vi "FL3001_simple.VI"() -> ()   [LabVIEW 2015]
uses:
  board.vis/Globals.vi
  board.vis/ESLSCDLL.dll
panel:
  in  "refresh display":bool
  in  "exit":bool
  in  "Trig Input Sel":string(combo)="I"
  out "meanB":dbl=197.0 format="%0#.1f"
  out "tRMSB":dbl format="%0#.1f"
  out "meanA":dbl=5347.758620689655 format="%0#.1f"
  in  "TRMS Pix":u32=400
  out "Signal Cam 2":u16[](graph)
  in  "extTrig":bool
  in  "ext. trig. slope":enum32{"1", "2", "3"}(radio)
  out "tRMSA":dbl=3.3455635332332063 format="%0#.1f"
  out "Measure ON":bool
  in  "no.of blocks (nob)":u32=1
  in  "block":u32(slide)=1 max=10 scale=0.9..1.0
  out "Signal Board 1 / Cam1":u16[](graph)=[0, 0, 0, 1, 0, 1, 0, 0, 5497, 8570, 8917, 9054, 9014, 9011, 8998, 9036, 9115, 9126, 9247, 9215, 9246, 9218, 9274, 9317, 9288, 9273, 9333, 9364, 9336, 9444, 9291, 9321, 9410, 9473, 9505, 9572, 9432, 9485, 9538, 9474, 9597, 9570, 9529, 9555, 9568, 9553, 9543, 9482, 9667, 9586, 9609, 9646, 9700, 9684, 9610, 9559, 9714, 9684, 9600, 9717, 9720, 9617, 9735, 9735, 9735, 9706, 9735, 9735, 9724, 9648, 9727, 9727, 9651, 9658, 9703, 9711, 9697, 9735, 9710, 9735, 9871, 9735, 9735, 9735, 9735, 9735, 9735, 9735, 9720, 9735, 9735, 9876, 9735, 9734, 9718, 9735, 9735, 9735, 9735, 9896, 9870, 9735, 9735, 9735, 9735, 9735, 9735, 9731, 9932, 9735, 9728, 9735, 9933, 9917, 9680, 9735, 9913, 9735, 9735, 9735, 9735, 9735, 9735, 9735, 9735, 9900, 9735, 9735, 9735, 9735, 9735, 9735, 9735, 9735, 9735, 9735, 9735, 9891, 9735, 9869, 9735, 9735, 9735, 9735, 9735, 9735, 9735, 9735, 9735, 9735, 9902, 9735, 9735, 9735, 9735, 9732, 9735, 9735, 9735, 9735, 9735, 9894, 9735, 9875, 9735, 9735, 9735, 9735, 9735, 9735, 9735, 9925, 9934, 9735, 9735, 9735, 9735, 9877, 9735, 9894, 9894, 9735, 9735, 9890, 9735, 9963, 9947, 9883, 9735, 9735, 9735, 9735, 9898, 9927, 9926, 9952, 9735, 9900, 9735, 9938, 9735, 9999, 9977, 9896, 9978, 9903, 9992, 9940, 9965, 9972, 9735, 9974, 9735, 9943, 9873, 9890, 9951, 9735, 9964, 9735, 9992, 9918, 10003, 9919, 9973, 9735, 9896, 9896, 9735, 9940, 10059, 9926, 9897, 9961, 9968, 9915, 9880, 9916, 9991, 9981, 9735, 9978, 10057, 10022, 9951, 9912, 9969, 10066, 9928, 9946, 9951, 10004, 9935, 9910, 9960, 9921, 9967, 9908, 10022, 9955, 9950, 9962, 9962, 9978, 10000, 9945, 9940, 9978, 9986, 10047, 10095, 9939, 10007, 9948, 10071, 10018, 10092, 10027, 10006, 10025, 10016, 10008, 10045, 10094, 10057, 10015, 9980, 10003, 10025, 10019, 10014, 10103, 10047, 9995, 9975, 10138, 9958, 10025, 9965, 10086, 10022, 9960, 10109, 10037, 10043, 10076, 10012, 10010, 10040, 10037, 10000, 9996, 10090, 10132, 10050, 10050, 9991, 10116, 10059, 10020, 9985, 10079, 10137, 10064, 10103, 10043, 10005, 10137, 10107, 10092, 10078, 10139, 10116, 10148, 10041, 10091, 10039, 10069, 10046, 10113, 10119, 10079, 10014, 10045, 10124, 10112, 10080, 10078, 10067, 10093, 10156, 10161, 10131, 10151, 10111, 10118, 10100, 10072, 10153, 10172, 10163, 10113, 10125, 10187, 10213, 10211, 10146, 10170, 10120, 10172, 10077, 10186, 10108, 10147, 10099, 10127, 10161, 10114, 10109, 10218, 10209, 10174, 10156, 10147, 10098, 10193, 10177, 10190, 10185, 10147, 10180, 10135, 10151, 10144, 10173, 10482, 10205, 10182, 10105, 10207, 10215, 10147, 10122, 10147, 10188, 10187, 10297, 10207, 10115, 10233, 10231, 10246, 10236, 10256, 10271, 10232, 10232, 10198, 10175, 10232, 10564, 10282, 10222, 10134, 10340, 10253, 10266, 10312, 10194, 10208, 10153, 10194, 10218, 10179, 10251, 10242, 10262, 10234, 10211, 10210, 10229, 10205, 10227, 10211, 10268, 10255, 10212, 10295, 10243, 10248, 10300, 10201, 10225, 10298, 10255, 10352, 10304, 10240, 10334, 10327, 10325, 10300, 10276, 10265, 10364, 10398, 10298, 10265, 10342, 10319, 10332, 10280, 10334, 10259, 10289, 10320, 10273, 10294, 10427, 10387, 10281, 10324, 10324, 10315, 10335, 10341, 10321, 10380, 10352, 10293, 10355, 10423, 10374, 10308, 10329, 10401, 10279, 11416, 10373, 10318, 10310, 10350, 10286, 10333, 10303, 10281, 10363, 10329, 10276, 10327, 10356, 10393, 10437, 10417, 10337, 10389, 10438, 10363, 10291, 10454, 10447, 10266, 10322, 10409, 10343, 10389, 10407, 10326, 10380, 10378, 10322, 10335, 10361, 10312, 10329, 10343, 10401, 10350, 10362, 10352, 10347, 10372, 10402, 10407, 10402, 10361, 10404, 10384, 10493, 10339, 10430, 10429, 10334, 10457, 10394, 10379, 10345, 10409, 10433, 10512, 10454, 10403, 10368, 10445, 10364, 10434, 10509, 10467, 10453, 10407, 10414, 10461, 10399, 10459, 10476, 10405, 10418, 10429, 10467, 10393, 10461, 10499, 10439, 10483, 10451, 10436, 10372, 10445, 10481, 10491, 10448, 10435, 10510, 10509, 10512, 10476, 10470, 10419, 10469, 10508, 10515, 10514, 10463, 10510, 10507, 10527, 10416, 10465, 10444, 10437, 10510, 10525, 10459, 10409, 10578, 10533, 10509, 10581, 10555, 10621, 10511, 10513, 10488, 10466, 10587, 10601, 10603, 10494, 10519, 10575, 10460, 10496, 10545, 10455, 10502, 10542, 10475, 10456, 10469, 10566, 10452, 10576, 10513, 10643, 10552, 10556, 10544, 10479, 10519, 10544, 10437, 10576, 10474, 10585, 10417, 10545, 10643, 10477, 10506, 10460, 10539, 10587, 10643, 10549, 10524, 10502, 10496, 10534, 10537, 10530, 10582, 10618, 10512, 10494, 10586, 10528, 10518, 10577, 10547, 10557, 10679, 10436, 10617, 10585, 10485, 10610, 10678, 10567, 10497, 10495, 10553, 10677, 10554, 10617, 10623, 10617, 10547, 10583, 10650, 10704, 10558, 10628, 10619, 10568, 10576, 10520, 10595, 10589, 10614, 10460, 10593, 10615, 10565, 10627, 10590, 10643, 10583, 10526, 10589, 10603, 10598, 10578, 10606, 10647, 10516, 10522, 10601, 10689, 10687, 10606, 10572, 10684, 10640, 10579, 10535, 10597, 10627, 10623, 10582, 10553, 10609, 10619, 10613, 10686, 10680, 10604, 10555, 10513, 10531, 10709, 10633, 10611, 10573, 10665, 10752, 10626, 10715, 10690, 10633, 10665, 10631, 10588, 10582, 10660, 10647, 10663, 10649, 10658, 10619, 10558, 10617, 10608, 10657, 10649, 10651, 10626, 10630, 10619, 10720, 10702, 10608, 10656, 10663, 10651, 10739, 10599, 10751, 10614, 10660, 10665, 10635, 10597, 10682, 10635, 10625, 10619, 10729, 10601, 10661, 10693, 10647, 10695, 10687, 10646, 10677, 10745, 10663, 10624, 10662, 10698, 10658, 10675, 10590, 10626, 10689, 10665, 10702, 10649, 10656, 10597, 10729, 10699, 10665, 10739, 10668, 10656, 10697, 10671, 10754, 10633, 10681, 10705, 10725, 10664, 10621, 10703, 10759, 10720, 10759, 10659, 10759, 10750, 10703, 10712, 10698, 10712, 10669, 10663, 10741, 10729, 10731, 10723, 10641, 10699, 10654, 10674, 10653, 10663, 10703, 10724, 10657, 10746, 10738, 10709, 10724, 10759, 10759, 10682, 10655, 10692, 10716, 10699, 10670, 10722, 10697, 10633, 10650, 10759, 10699, 10672, 10755, 10726, 10753, 10664, 10630, 10712, 10697, 10720, 10759, 10744, 10704, 10759, 10721, 10661, 10747, 10656, 10680, 10645, 10671, 10716, 10647, 10709, 10738, 10756, 10683, 10650, 10656, 10605, 10557, 10656, 10638, 10597, 10587, 10589, 10596, 10551, 10586, 10613, 10549, 10648, 10610, 10570, 10644, 10618, 10658, 10588, 10583, 10591, 10618, 10599, 10492, 10557, 10493, 10465, 10580, 10506, 10559, 10531, 10541, 10518, 10495, 10514, 10612, 10520, 10539, 10503, 10568, 10606, 10536, 10503, 10525, 10512, 10524, 10471, 10493, 10519, 10619, 10517, 10491, 10560, 10479, 10575, 10449, 10491, 10502, 10527, 10519, 10465, 10521, 10457, 10404, 10530, 10450, 10445, 10454, 10491, 10424, 10471, 10480, 10435, 10423, 10556, 10465, 10497, 10507, 10400, 10511, 10498, 10429, 10429, 10548, 10503, 10437, 10482, 10473, 10435, 10423, 10438, 10414, 10409, 10345, 10391, 10570, 10351, 10411, 10503, 10555, 10309, 10345, 10368, 10407, 10394, 10398, 10418, 10394, 10348, 10377, 10290, 10358, 10383, 10359, 10398, 10280, 10223, 10349, 10302, 10359, 10281, 10282, 10260, 10188, 10223, 10184, 10210, 10173, 10175, 10143, 10053, 10065, 10066, 10009, 10013, 9955, 9944, 9883, 5845, 5634, 5619, 5774, 5415, 5385, 5374, 5370, 5361, 5366, 5361, 5359, 5363, 5356, 5359, 5362, 5357, 5358, 5359, 5358, 5357, 5355, 5363, 5369, 5359, 5359, 5361, 5362, 5362, 5361, 5363, 5362, 5359, 5365, 5358, 5366, 5364, 5356, 5356, 5360, 5359, 5363, 5362]
  out "FREE \nRAM MB":dbl=28847.8671875
  out "BUILT-IN\nRAM MB":dbl=32640.29296875
  out "SEC":dbl=1.0
  out "MB RAM":dbl=2.0751953125
  in  "DAT in 10ns":u32
  in  "start":bool
  in  "sample":u32(slide)=1 max=3000 scale=0.9..1000.0
  in  "no.of samples (nos)":u32=1000
  in  "exposuretime[ms]":dbl=1.0 format="%.3f"
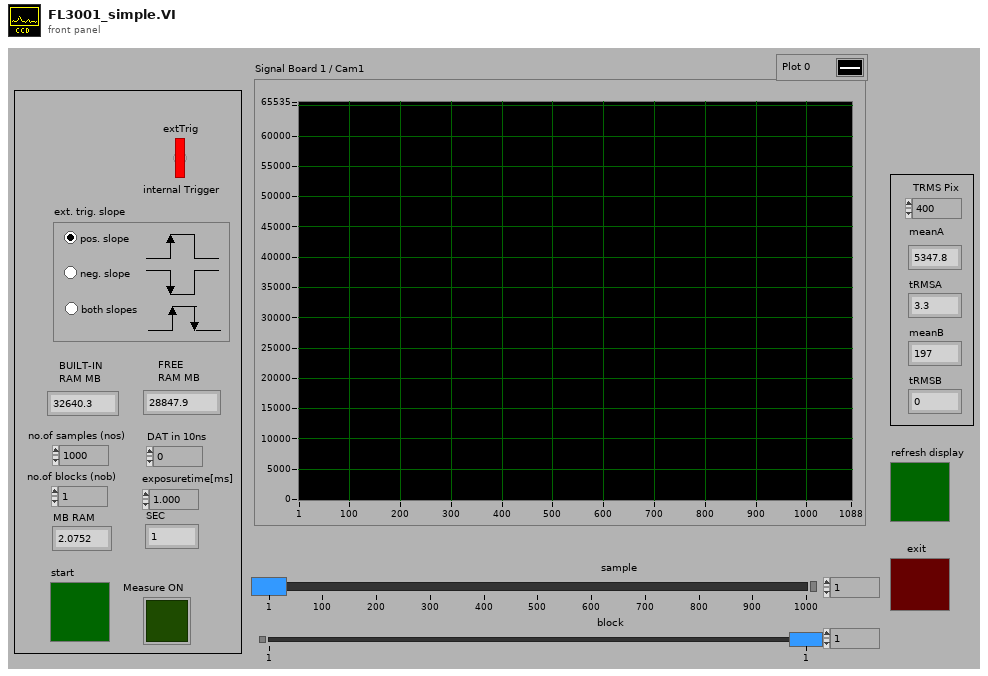
[diagram p1: front panel]
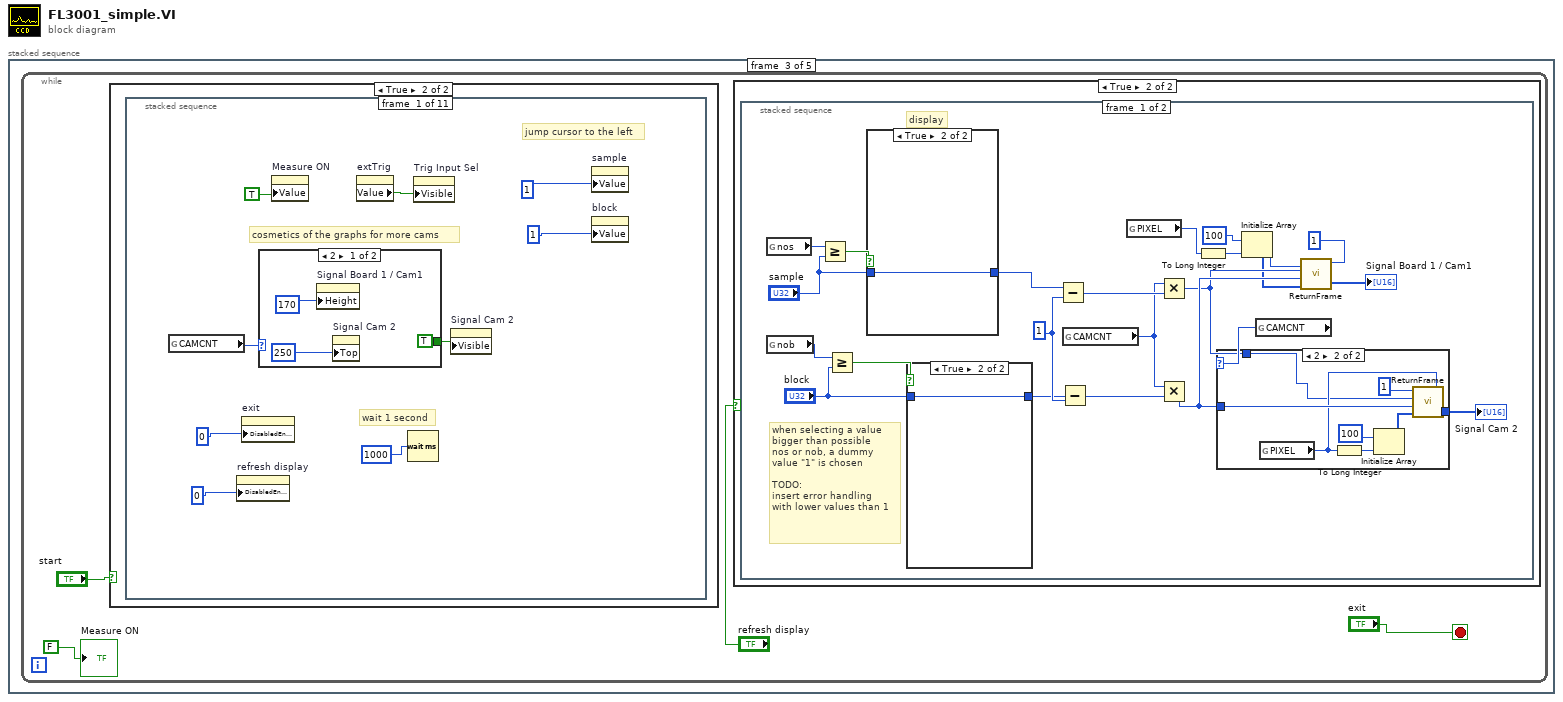
[diagram p0: block diagram]
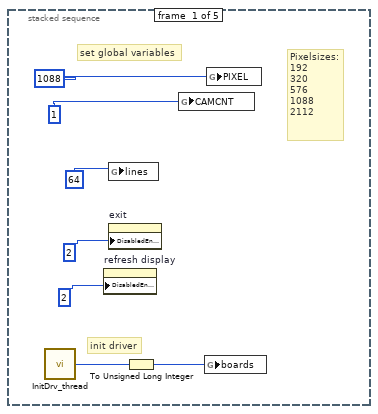
[diagram p2: hidden frame]
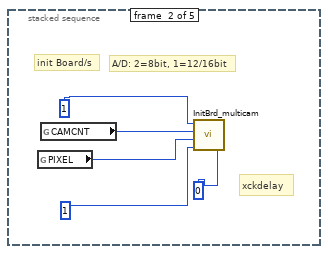
[diagram p3: hidden frame]
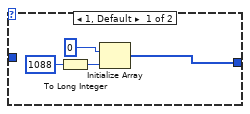
[diagram p5: hidden frame]
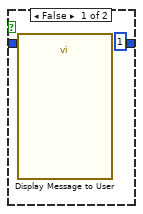
[diagram p6: hidden frame]
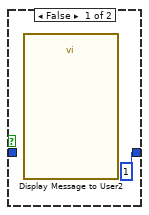
[diagram p7: hidden frame]
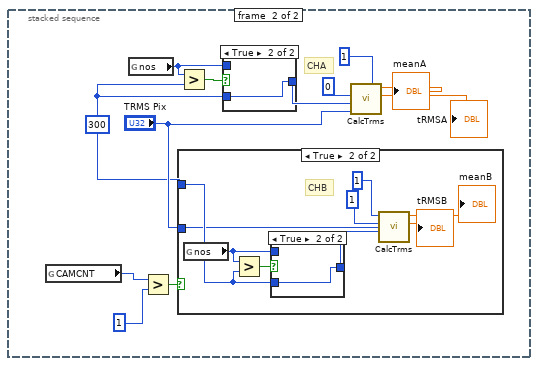
[diagram p8: hidden frame]
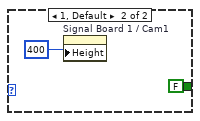
[diagram p13: hidden frame]
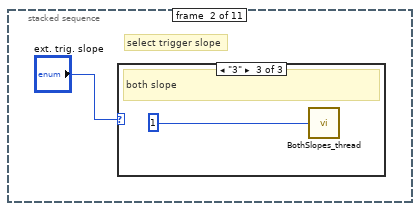
[diagram p14: hidden frame]
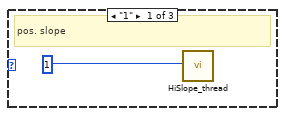
[diagram p15: hidden frame]
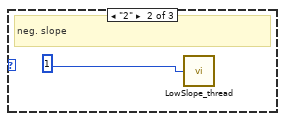
[diagram p16: hidden frame]
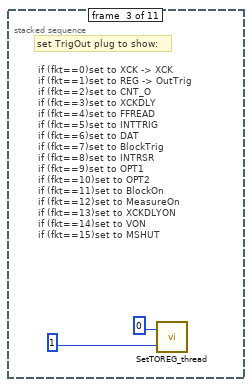
[diagram p17: hidden frame]
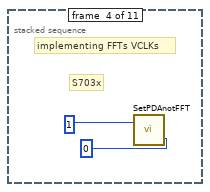
[diagram p18: hidden frame]
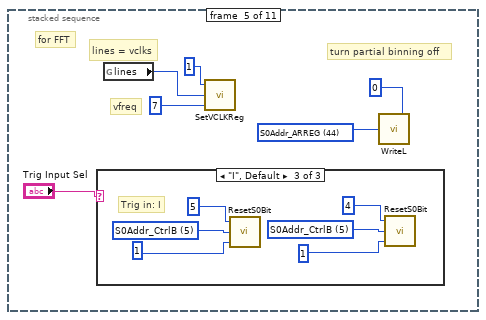
[diagram p19: hidden frame]
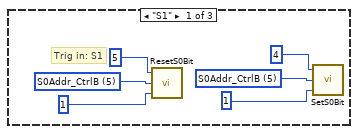
[diagram p20: hidden frame]
diagram:
  n1 = stacked-sequence {
    frame #0 {
      # "Pixelsizes:\n192\n320\n576\n1088\n2112"
      # "set global variables"
      # "init driver"
      n2 = call "InitDrv_thread.vi"() -> ("Boards"=w5:u8)  [unwired: 1 in]
      n3 = property on="refresh display" class="Bool (strict)"("DisabledEnum"=u16 2) -> ()  [unwired: 2 in, 2 out]
      n4 = global write "Globals.vi" "lines"(u32 64) -> ()
      n5 = property on="exit" class="Bool (strict)"("DisabledEnum"=u16 2) -> ()  [unwired: 2 in, 2 out]
      n6 = To Unsigned Long Integer(number=w5) -> (unsigned 32bit integer=w4:u32)
      n7 = global write "Globals.vi" "CAMCNT"(u32 1) -> ()
      n8 = global write "Globals.vi" "boards"(w4) -> ()
      n9 = global write "Globals.vi" "PIXEL"(u32 1088) -> ()
    }
    frame #1 {
      # "xckdelay"
      # "init Board/s"
      # "A/D: 2=8bit, 1=12/16bit"
      n10 = global read "Globals.vi" "PIXEL"() -> (w10:u32)
      n11 = global read "Globals.vi" "CAMCNT"() -> (w12:u32)
      n12 = call "InitBrd_multicam.vi"("xckdly"=u32 0, "flag816"=u32 1, "pixel"=w10, "camcnt"=w12, "board_sel"=u32 1) -> ()  [unwired: 2 in]
    }
    frame #2 {
      n13 = while {
        stop <- "exit" stop-if-true
        n14 = case shown="True" "start" {
          frame False {
          }
          frame True {
            n15 = stacked-sequence {
              frame #0 {
                # "wait 1 second"
                # "jump cursor to the left"
                # "cosmetics of the graphs for more cams"
                n16 = global read "Globals.vi" "CAMCNT"() -> (w87:u32)
                n17 = property on="refresh display" class="Bool (strict)"("DisabledEnum"=u16 0) -> ()  [unwired: 2 in, 2 out]
                n18 = property on="exit" class="Bool (strict)"("DisabledEnum"=u16 0) -> ()  [unwired: 2 in, 2 out]
                n19 = case shown="2" w87 {
                  tunnel: [TRUE FALSE] -> w88
                  frame 2 {
                    n20 = property on="Signal Board 1 / Cam1" class="WFGraph (strict)"("Height"=u32 170) -> ()  [unwired: 2 in, 2 out]
                    n21 = property on="Signal Cam 2" class="WFGraph (strict)"("Top"=250) -> ()  [unwired: 2 in, 2 out]
                  }
                  frame 1, Default {
                    n22 = property on="Signal Board 1 / Cam1" class="WFGraph (strict)"("Height"=u32 400) -> ()  [unwired: 2 in, 2 out]
                  }
                }
                n23 = property on="Measure ON" class="Bool (strict)"("Value"=TRUE) -> ()  [unwired: 2 in, 2 out]
                n24 = property on="extTrig" class="Bool (strict)"() -> ("Value"=w85:bool)  [unwired: 2 in, 2 out]
                n25 = Wait (ms)(milliseconds to wait=u16 1000) -> ()  [unwired: 1 out]
                n26 = property on="Trig Input Sel" class="CmbBox"("Visible"=w85) -> ()  [unwired: 2 in, 2 out]
                n27 = property on="Signal Cam 2" class="WFGraph (strict)"("Visible"=w88) -> ()  [unwired: 2 in, 2 out]
                n28 = property on="sample" class="Slide (strict)"("Value"=u32 1) -> ()  [unwired: 2 in, 2 out]
                n29 = property on="block" class="Slide (strict)"("Value"=u32 1) -> ()  [unwired: 2 in, 2 out]
              }
              frame #1 {
                # "select trigger slope"
                n30 = case shown="\"3\"" "ext. trig. slope" {
                  frame "1" {
                    # "pos. slope"
                    n31 = call "HiSlope_thread.vi"("board_sel"=u32 1) -> ()  [unwired: 1 in]
                  }
                  frame "2" {
                    # "neg. slope"
                    n32 = call "LowSlope_thread.vi"("board_sel"=u32 1) -> ()  [unwired: 1 in]
                  }
                  frame "3" {
                    # "both slope"
                    n33 = call "BothSlopes_thread.vi"("board_sel"=u32 1) -> ()  [unwired: 1 in]
                  }
                }
              }
              frame #2 {
                # "if (fkt==0)set to XCK -> XCK\nif (fkt==1)set to REG -> OutTrig\nif (fkt==2)set to CNT_O\nif (fkt==3)set to XCKDLY\nif (fkt==4)set to FFREAD\nif (fkt==5)set to INTTRIG\nif (fkt==6)set to DAT\nif (fkt==7)set to BlockTrig\nif (fkt==8)set to INTRSR\nif (fkt==9)set to OPT1\nif (fkt==10)set to OPT2\nif (fkt==11)set to BlockOn\nif (fkt==12)set to MeasureOn\nif (fkt==13)set to XCKDLYON \nif (fkt==14)set to VON         \nif (fkt==15)set to MSHUT"
                # "set TrigOut plug to show:"
                n34 = call "SetTOREG_thread.vi"("board_sel"=u32 1, "fkt"=u8 0) -> ()  [unwired: 1 in]
              }
              frame #3 {
                # "S703x"
                # "implementing FFTs VCLKs"
                n35 = call "SetPDAnotFFT.vi"("set"=u8 0, "board_sel"=u32 1) -> ()  [unwired: 1 in]
              }
              frame #4 {
                w105 = u8 44 items=["S0Addr_CtrlA"=4, "S0Addr_CtrlB"=5, "S0Addr_CtrlC"=6, "S0Addr_XCKLL"=8, "S0Addr_XCKLH"=9, "S0Addr_XCKHL"=10, "S0Addr_XCKMSB"=11, "S0Addr_XCKCNTLL"=12, "S0Addr_XCKCNTLH"=13, "S0Addr_XCKCNTHL"=14, "S0Addr_XCKCNTMSB"=15, "S0Addr_PIXREGlow"=16, "S0Addr_PIXREGhigh"=17, "S0Addr_FREQREG"=18, "S0Addr_FF_FLAGS"=19, "S0Addr_FIFOCNT"=20, "S0Addr_VCLKCTRL"=24, "S0Addr_EBST"=28, "S0Addr_DAT"=32, "S0Addr_EC"=36, "S0Addr_TOR"=40, "S0Addr_ARREG"=44, "S0Addr_GIOREG"=48, "S0Addr_DELAYEC"=52, "S0Addr_IRQREG"=56, "S0Addr_PCI"=60]
                # "turn partial binning off"
                # "vfreq"
                # "lines = vclks"
                # "for FFT"
                n36 = case shown="\"I\", Default" "Trig Input Sel" {
                  frame "S1" {
                    w113 = u8 5 items=["S0Addr_CtrlA"=4, "S0Addr_CtrlB"=5, "S0Addr_CtrlC"=6, "S0Addr_XCKLL"=8, "S0Addr_XCKLH"=9, "S0Addr_XCKHL"=10, "S0Addr_XCKMSB"=11, "S0Addr_XCKCNTLL"=12, "S0Addr_XCKCNTLH"=13, "S0Addr_XCKCNTHL"=14, "S0Addr_XCKCNTMSB"=15, "S0Addr_PIXREGlow"=16, "S0Addr_PIXREGhigh"=17, "S0Addr_FREQREG"=18, "S0Addr_FF_FLAGS"=19, "S0Addr_FIFOCNT"=20, "S0Addr_VCLKCTRL"=24, "S0Addr_EBST"=28, "S0Addr_DAT"=32, "S0Addr_EC"=36, "S0Addr_TOR"=40, "S0Addr_ARREG"=44, "S0Addr_GIOREG"=48, "S0Addr_DELAYEC"=52, "S0Addr_IRQREG"=56, "S0Addr_PCI"=60]
                    w110 = u8 5 items=["S0Addr_CtrlA"=4, "S0Addr_CtrlB"=5, "S0Addr_CtrlC"=6, "S0Addr_XCKLL"=8, "S0Addr_XCKLH"=9, "S0Addr_XCKHL"=10, "S0Addr_XCKMSB"=11, "S0Addr_XCKCNTLL"=12, "S0Addr_XCKCNTLH"=13, "S0Addr_XCKCNTHL"=14, "S0Addr_XCKCNTMSB"=15, "S0Addr_PIXREGlow"=16, "S0Addr_PIXREGhigh"=17, "S0Addr_FREQREG"=18, "S0Addr_FF_FLAGS"=19, "S0Addr_FIFOCNT"=20, "S0Addr_VCLKCTRL"=24, "S0Addr_EBST"=28, "S0Addr_DAT"=32, "S0Addr_EC"=36, "S0Addr_TOR"=40, "S0Addr_ARREG"=44, "S0Addr_GIOREG"=48, "S0Addr_DELAYEC"=52, "S0Addr_IRQREG"=56, "S0Addr_PCI"=60]
                    # "Trig in: S1"
                    n37 = call "ResetS0Bit.vi"("drv"=u32 1, "Address"=w110, "bitnumber"=u32 5) -> ()
                    n38 = call "SetS0Bit.vi"("board_sel"=u32 1, "Address"=w113, "bitnumber"=u32 4) -> ()
                  }
                  frame "S2" {
                    w116 = u8 5 items=["S0Addr_CtrlA"=4, "S0Addr_CtrlB"=5, "S0Addr_CtrlC"=6, "S0Addr_XCKLL"=8, "S0Addr_XCKLH"=9, "S0Addr_XCKHL"=10, "S0Addr_XCKMSB"=11, "S0Addr_XCKCNTLL"=12, "S0Addr_XCKCNTLH"=13, "S0Addr_XCKCNTHL"=14, "S0Addr_XCKCNTMSB"=15, "S0Addr_PIXREGlow"=16, "S0Addr_PIXREGhigh"=17, "S0Addr_FREQREG"=18, "S0Addr_FF_FLAGS"=19, "S0Addr_FIFOCNT"=20, "S0Addr_VCLKCTRL"=24, "S0Addr_EBST"=28, "S0Addr_DAT"=32, "S0Addr_EC"=36, "S0Addr_TOR"=40, "S0Addr_ARREG"=44, "S0Addr_GIOREG"=48, "S0Addr_DELAYEC"=52, "S0Addr_IRQREG"=56, "S0Addr_PCI"=60]
                    w118 = u8 5 items=["S0Addr_CtrlA"=4, "S0Addr_CtrlB"=5, "S0Addr_CtrlC"=6, "S0Addr_XCKLL"=8, "S0Addr_XCKLH"=9, "S0Addr_XCKHL"=10, "S0Addr_XCKMSB"=11, "S0Addr_XCKCNTLL"=12, "S0Addr_XCKCNTLH"=13, "S0Addr_XCKCNTHL"=14, "S0Addr_XCKCNTMSB"=15, "S0Addr_PIXREGlow"=16, "S0Addr_PIXREGhigh"=17, "S0Addr_FREQREG"=18, "S0Addr_FF_FLAGS"=19, "S0Addr_FIFOCNT"=20, "S0Addr_VCLKCTRL"=24, "S0Addr_EBST"=28, "S0Addr_DAT"=32, "S0Addr_EC"=36, "S0Addr_TOR"=40, "S0Addr_ARREG"=44, "S0Addr_GIOREG"=48, "S0Addr_DELAYEC"=52, "S0Addr_IRQREG"=56, "S0Addr_PCI"=60]
                    # "Trig in: S2"
                    n39 = call "SetS0Bit.vi"("board_sel"=u32 1, "Address"=w118, "bitnumber"=u32 5) -> ()
                    n40 = call "ResetS0Bit.vi"("drv"=u32 1, "Address"=w116, "bitnumber"=u32 4) -> ()
                  }
                  frame "I", Default {
                    w125 = u8 5 items=["S0Addr_CtrlA"=4, "S0Addr_CtrlB"=5, "S0Addr_CtrlC"=6, "S0Addr_XCKLL"=8, "S0Addr_XCKLH"=9, "S0Addr_XCKHL"=10, "S0Addr_XCKMSB"=11, "S0Addr_XCKCNTLL"=12, "S0Addr_XCKCNTLH"=13, "S0Addr_XCKCNTHL"=14, "S0Addr_XCKCNTMSB"=15, "S0Addr_PIXREGlow"=16, "S0Addr_PIXREGhigh"=17, "S0Addr_FREQREG"=18, "S0Addr_FF_FLAGS"=19, "S0Addr_FIFOCNT"=20, "S0Addr_VCLKCTRL"=24, "S0Addr_EBST"=28, "S0Addr_DAT"=32, "S0Addr_EC"=36, "S0Addr_TOR"=40, "S0Addr_ARREG"=44, "S0Addr_GIOREG"=48, "S0Addr_DELAYEC"=52, "S0Addr_IRQREG"=56, "S0Addr_PCI"=60]
                    w122 = u8 5 items=["S0Addr_CtrlA"=4, "S0Addr_CtrlB"=5, "S0Addr_CtrlC"=6, "S0Addr_XCKLL"=8, "S0Addr_XCKLH"=9, "S0Addr_XCKHL"=10, "S0Addr_XCKMSB"=11, "S0Addr_XCKCNTLL"=12, "S0Addr_XCKCNTLH"=13, "S0Addr_XCKCNTHL"=14, "S0Addr_XCKCNTMSB"=15, "S0Addr_PIXREGlow"=16, "S0Addr_PIXREGhigh"=17, "S0Addr_FREQREG"=18, "S0Addr_FF_FLAGS"=19, "S0Addr_FIFOCNT"=20, "S0Addr_VCLKCTRL"=24, "S0Addr_EBST"=28, "S0Addr_DAT"=32, "S0Addr_EC"=36, "S0Addr_TOR"=40, "S0Addr_ARREG"=44, "S0Addr_GIOREG"=48, "S0Addr_DELAYEC"=52, "S0Addr_IRQREG"=56, "S0Addr_PCI"=60]
                    # "Trig in: I"
                    n41 = call "ResetS0Bit.vi"("drv"=u32 1, "Address"=w125, "bitnumber"=u32 5) -> ()
                    n42 = call "ResetS0Bit.vi"("drv"=u32 1, "Address"=w122, "bitnumber"=u32 4) -> ()
                  }
                }
                n43 = global read "Globals.vi" "lines"() -> (w107:u32)
                n44 = call "SetVCLKReg.vi"("vfreq"=u8 7, "lines"=w107, "board_sel"=u32 1) -> ()  [unwired: 1 in]
                n45 = call "WriteL.vi"("val"=u32 0, "offset"=w105) -> ()
              }
              frame #5 {
                w127 = u16 1  # is_fft
                w130 = u16 0  # trigger
                # "select VCLK ON\n0 for VCLK off\n1 for VCLK on"
                # "set trigger input\ntrigger = x0 XCK\ntrigger = x1 EXTTRIG\ntrigger = x2 DAT"
                # "init routine for 3001"
                n46 = global read "Globals.vi" "PIXEL"() -> (w128:u32)
                n47 = To Unsigned Word Integer(number=w128) -> (unsigned 16bit integer=w129:u16)
                n48 = dll-call lib="C:/ENTW/PCIE/lv64/board.vis/ESLSCDLL.dll" fn="DLLInitCamera3001" ("lwlscdll.dll:DLLSetADAmpRed")("drv"=u32 1, "pixel"=w129, "trigger_input"=w130, "is_fft"=w127) -> ()  [unwired: 8 in, 2 out]
              }
              frame #6 {
                # "bit31 must be set for enabling DAT(add 0x80000000) to REG 0x20"
                # "is only valid for external trigger!"
                # "this examples shows how to set the DAT (delay after trigger)"
                n49 = Equal To 0?(x="DAT in 10ns") -> (x = 0?=w132:bool)
                n50 = case shown="True" w132 {
                  tunnel: "DAT in 10ns" -> [w136 _]
                  frame False {
                    w134 = u8 32 items=["S0Addr_CtrlA"=4, "S0Addr_CtrlB"=5, "S0Addr_CtrlC"=6, "S0Addr_XCKLL"=8, "S0Addr_XCKLH"=9, "S0Addr_XCKHL"=10, "S0Addr_XCKMSB"=11, "S0Addr_XCKCNTLL"=12, "S0Addr_XCKCNTLH"=13, "S0Addr_XCKCNTHL"=14, "S0Addr_XCKCNTMSB"=15, "S0Addr_PIXREGlow"=16, "S0Addr_PIXREGhigh"=17, "S0Addr_FREQREG"=18, "S0Addr_FF_FLAGS"=19, "S0Addr_FIFOCNT"=20, "S0Addr_VCLKCTRL"=24, "S0Addr_EBST"=28, "S0Addr_DAT"=32, "S0Addr_EC"=36, "S0Addr_TOR"=40, "S0Addr_ARREG"=44, "S0Addr_GIOREG"=48, "S0Addr_DELAYEC"=52, "S0Addr_IRQREG"=56, "S0Addr_PCI"=60]
                    n51 = Add(x=u32 2147483648, y=w136) -> (x+y=w135:u32)
                    n52 = call "WriteL_thread.vi"("val"=w135, "board_sel"=u32 1, "offset"=w134) -> ()
                  }
                  frame True {
                    w139 = u8 32 items=["S0Addr_CtrlA"=4, "S0Addr_CtrlB"=5, "S0Addr_CtrlC"=6, "S0Addr_XCKLL"=8, "S0Addr_XCKLH"=9, "S0Addr_XCKHL"=10, "S0Addr_XCKMSB"=11, "S0Addr_XCKCNTLL"=12, "S0Addr_XCKCNTLH"=13, "S0Addr_XCKCNTHL"=14, "S0Addr_XCKCNTMSB"=15, "S0Addr_PIXREGlow"=16, "S0Addr_PIXREGhigh"=17, "S0Addr_FREQREG"=18, "S0Addr_FF_FLAGS"=19, "S0Addr_FIFOCNT"=20, "S0Addr_VCLKCTRL"=24, "S0Addr_EBST"=28, "S0Addr_DAT"=32, "S0Addr_EC"=36, "S0Addr_TOR"=40, "S0Addr_ARREG"=44, "S0Addr_GIOREG"=48, "S0Addr_DELAYEC"=52, "S0Addr_IRQREG"=56, "S0Addr_PCI"=60]
                    n53 = call "WriteL_thread.vi"("val"=u32 0, "board_sel"=u32 1, "offset"=w139) -> ()
                  }
                }
              }
              frame #7 {
                # "set EC"
                # "calculation of MB RAM an SEC and setting scale max"
                # "MB"
                # "ushort"
                n54 = global read "Globals.vi" "PIXEL"() -> (w167:u32)
                n55 = global read "Globals.vi" "nob"() -> (w148:u32)
                n56 = global read "Globals.vi" "nos"() -> (w150:u32)
                n57 = Multiply(x="no.of samples (nos)", y=w167) -> (x*y=w165:u32)
                n58 = To Double Precision Float(number=w150) -> (double precision float=w149:dbl)
                n59 = To Double Precision Float(number=w148) -> (double precision float=w147:dbl)
                n60 = Multiply(x=w165, y=u32 2) -> (x*y=w146:u32)
                n61 = global read "Globals.vi" "boards"() -> (w166:u32)
                n62 = global read "Globals.vi" "CAMCNT"() -> (w145:u32)
                n63 = call "ResetEC.vi"("board_sel"=u32 1) -> ()  [unwired: 2 in]
                n64 = property on="sample" class="Slide (strict)"("Scale.Maximum"=w149) -> ()  [unwired: 2 in, 2 out]
                n65 = property on="block" class="Slide (strict)"("Scale.Maximum"=w147) -> ()  [unwired: 2 in, 2 out]
                n66 = To Unsigned Long Integer(number=w145) -> (unsigned 32bit integer=w144:u32)
                n67 = Multiply(x=w144, y=w146) -> (x*y=w143:u32)
                n68 = Multiply(x=w143, y=w166) -> (x*y=w156:u32)
                n69 = To Double Precision Float(number=w156) -> (double precision float=w155:dbl)
                n70 = Divide(x=w155, y=1048576.0) -> (x/y=w158:dbl)
                n71 = To Double Precision Float(number="no.of blocks (nob)") -> (double precision float=w153:dbl)
                n72 = Multiply(x=w158, y=w153) -> (x*y=→"MB RAM":dbl)
                n73 = global write "Globals.vi" "nos"("no.of samples (nos)") -> ()
                n74 = Multiply(x="no.of samples (nos)", y="no.of blocks (nob)") -> (x*y=w151:u32)
                n75 = global write "Globals.vi" "nob"("no.of blocks (nob)") -> ()
                n76 = To Double Precision Float(number=w151) -> (double precision float=w152:dbl)
                n77 = global write "Globals.vi" "exp time"("exposuretime[ms]") -> ()
                n78 = Multiply(x="exposuretime[ms]", y=w152) -> (x*y=w164:dbl)
                n79 = Divide(x=w164, y=1000.0) -> (x/y=→"SEC":dbl)
              }
              frame #8 {
                n80 = call "FreeMemInfo.vi"() -> ("PhysicalSpace"=→"BUILT-IN\nRAM MB":dbl, "PhysicalFreeSpace"=→"FREE \nRAM MB":dbl)  [unwired: 1 in]
              }
              frame #9 {
                # "Setup DMA"
                n81 = global read "Globals.vi" "nos"() -> (w172:u32)
                n82 = global read "Globals.vi" "nob"() -> (w171:u32)
                n83 = call "SetupDMA_thread.vi"("blocks"=w171, "nos"=w172, "Board_sel"=u32 1) -> ()  [unwired: 2 in]
              }
              frame #10 {
                # "ext. block trig\n0: internal: Space\n1: PCI \"I\"\n2: S1\n3: S2"
                # "block trigger (depreciated, keep 0)\n0: internal -> next block is started immediately \n1: external -> all blocks on one trigger (via DLL)\n2: external -> one block per trigger (via DLL)"
                # "start measurement"
                n84 = global read "Globals.vi" "exp time"() -> (w176:dbl)
                n85 = Multiply(x=1000.0, y=w176) -> (x*y=w174:dbl)
                n86 = To Unsigned Long Integer(number=w174) -> (unsigned 32bit integer=w181:u32)
                n87 = case shown="True" "extTrig" {
                  tunnel: [u8 0 u8 1] -> w179
                  frame False {
                  }
                  frame True {
                  }
                }
                n88 = call "ReadFFLoop_thread.vi"("board_sel"=u32 1, "exptus"=w181, "ExtTrig"=w179, "btrig_ch"=u8 3, "blocktrigger"=u8 0) -> ()
              }
            }
          }
        }
        n89 = case shown="True" "refresh display" {
          frame False {
          }
          frame True {
            n90 = stacked-sequence {
              frame #0 {
                w38 = u32 1
                # "when selecting a value\nbigger than possible\nnos or nob, a dummy \nvalue \"1\" is chosen\n\nTODO:\ninsert error handling\nwith lower values than 1"
                # "display"
                n91 = global read "Globals.vi" "nos"() -> (w37:u32)
                n92 = global read "Globals.vi" "nob"() -> (w32:u32)
                n93 = Greater Or Equal?(x=w37, y="sample") -> (x >= y?=w30:bool)
                n94 = Greater Or Equal?(x=w32, y="block") -> (x >= y?=w29:bool)
                n95 = case shown="True" w30 {
                  tunnel: [u32 1 w54] -> w36
                  tunnel: "sample" -> [_ w54]
                  frame False {
                    n96 = call "Display Message to User2"() -> ()  [unwired: 10 in, 2 out]
                  }
                  frame True {
                  }
                }
                n97 = case shown="True" w29 {
                  tunnel: [u32 1 w52] -> w34
                  tunnel: "block" -> [_ w52]
                  frame False {
                    n98 = call "Display Message to User"() -> ()  [unwired: 10 in, 2 out]
                  }
                  frame True {
                  }
                }
                n99 = Subtract(x=w36, y=w38) -> (x-y=w28:u32)
                n100 = Subtract(x=w34, y=w38) -> (x-y=w24:u32)
                n101 = global read "Globals.vi" "CAMCNT"() -> (w17:u32)
                n102 = global read "Globals.vi" "PIXEL"() -> (w23:u32)
                n103 = Multiply(x=w17, y=w28) -> (x*y=w26:u32)
                n104 = Multiply(x=w17, y=w24) -> (x*y=w27:u32)
                n105 = To Long Integer(number=w23) -> (32bit integer=w22:i32)
                n106 = Initialize Array(u16 100, w22) -> (w18:u16[])
                n107 = global read "Globals.vi" "CAMCNT"() -> (w31:u32)
                n108 = case shown="2" w31 {
                  tunnel: w27 -> [_ w47]
                  tunnel: w26 -> [_ w43]
                  tunnel: [w39 w44] -> w25
                  frame 1, Default {
                    n109 = To Long Integer(number=u16 1088) -> (32bit integer=w40:i32)
                    n110 = Initialize Array(u16 0, w40) -> (w39:u16[])
                  }
                  frame 2 {
                    n111 = global read "Globals.vi" "PIXEL"() -> (w45:u32)
                    n112 = To Long Integer(number=w45) -> (32bit integer=w46:i32)
                    n113 = Initialize Array(u16 100, w46) -> (w48:u16[])
                    n114 = call "ReturnFrame.vi"("length"=w45, "Data Values In"=w48, "curr_nob"=w47, "curr_nos"=w43, "Drv"=u32 1) -> ("Data Values Out"=w44:u16[])
                  }
                }
                "Signal Cam 2" <- w25
                n115 = call "ReturnFrame.vi"("length"=w23, "Data Values In"=w18, "curr_nob"=w27, "curr_nos"=w26, "Drv"=u32 1) -> ("Data Values Out"=→"Signal Board 1 / Cam1":u16[])
              }
              frame #1 {
                w61 = u32 300
                # "CHA"
                n116 = global read "Globals.vi" "CAMCNT"() -> (w63:u32)
                n117 = global read "Globals.vi" "nos"() -> (w57:u32)
                n118 = Greater?(x=w63, y=u32 1) -> (0:w65:bool)
                n119 = case shown="True" w65 {
                  tunnel: w61 -> [_ w70]
                  tunnel: "TRMS Pix" -> [_ w69]
                  frame False {
                  }
                  frame True {
                    # "CHB"
                    n120 = global read "Globals.vi" "nos"() -> (w73:u32)
                    n121 = Greater?(x=w73, y=w70) -> (0:w75:bool)
                    n122 = case shown="True" w75 {
                      tunnel: [w76 w77] -> w74
                      tunnel: w70 -> [_ w77]
                      tunnel: w73 -> [w76 _]
                      frame False {
                      }
                      frame True {
                      }
                    }
                    n123 = call "CalcTrms.vi"("TRMSpix"=w69, "scans"=w74, "CAMpos"=u16 1, "board_sel"=u32 1) -> ("TRMS 1"=→"tRMSB":dbl, "mean 1"=→"meanB":dbl)  [unwired: 2 out]
                  }
                }
                n124 = Greater?(x=w57, y=w61) -> (0:w55:bool)
                n125 = case shown="True" w55 {
                  tunnel: [w78 w79] -> w56
                  tunnel: w61 -> [_ w79]
                  tunnel: w57 -> [w78 _]
                  frame False {
                  }
                  frame True {
                  }
                }
                n126 = call "CalcTrms.vi"("TRMSpix"="TRMS Pix", "scans"=w56, "CAMpos"=0, "board_sel"=u32 1) -> ("TRMS 1"=→"tRMSA":dbl, "mean 1"=→"meanA":dbl)  [unwired: 2 out]
              }
            }
          }
        }
        "Measure ON" <- FALSE
      }
    }
    frame #3 {
      n127 = call "FFStop.vi"() -> ()  [unwired: 1 in]
    }
    frame #4 {
      # "exit"
      # "do not omit, or next call of driver will go wrong."
      n128 = call "Exit.vi"("board_sel"=u32 1) -> ()  [unwired: 1 in]
    }
  }
